vi "1D_array_from_binary_data.vi"(5 "little-endian?":bool, 7 "inputArray(type)":variant, 8 "error in (no error)":errorcluster, 11 "byteArray":u8[](array[numeric])) -> (0 "error out":errorcluster, 3 "dataArray":variant)   [LabVIEW 2015, in "BSON_convertors_Library.lvlib"]
uses:
  BSON_convertors_Library.lvlib
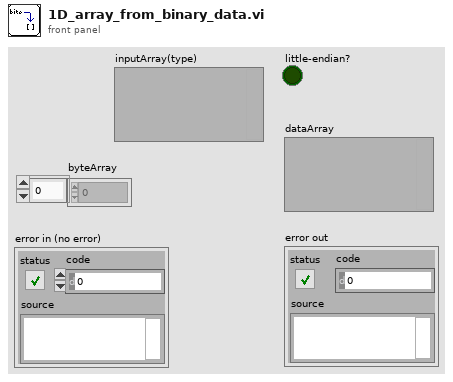
[diagram p1: front panel]
types:
  T1 = enum16{"big-endian, network order", "native, host order", "little-endian"}
  T2 = typedef "Type Descriptor Enumeration__ogtk.ctl" = enum8{"<Null>", "I8", "I16", "I32", "I64", "U8", "U16", "U32", "U64", "SGL", "DBL", "EXT", "CSG", "CDB", "CXT", "0x0F", "0x10", "0x11", "0x12", "0x13", "0x14", "Enum U8", "Enum U16", "Enum U32", "Enum U64", "SGL PQ", "DBL PQ", "EXT PQ", "CSG PQ", "CDB PQ", "CXT PQ", "0x1F", "0x20", "Boolean", "0x22", "0x23", "0x24", "0x25", "0x26", "0x27", "0x28", "0x29", "0x2A", "0x2B", "0x2C", "0x2D", "0x2E", "0x2F", "String", "0x31", "Path", "Pict", "0x34", "0x35", "0x36", "DAQ", "0x38", "0x39", "0x3A", "0x3B", "0x3C", "0x3D", "0x3E", "0x3F", "Array", "0x41", "0x42", "0x43", "0x44", "0x45", "0x46", "0x47", "0x48", "0x49", "0x4A", "0x4B", "0x4C", "0x4D", "0x4E", "0x4F", "Cluster", "0x51", "0x52", "Variant", "Waveform", "0x55", "0x56", "0x57", "0x58", "0x59", "0x5A", "0x5B", "0x5C", "0x5D", "0x5E", "0x5F", "0x60", "0x61", "0x62", "0x63", "0x64", "0x65", "0x66", "0x67", "0x68", "0x69", "0x6A", "0x6B", "0x6C", "0x6D", "0x6E", "0x6F", "Refnum"}
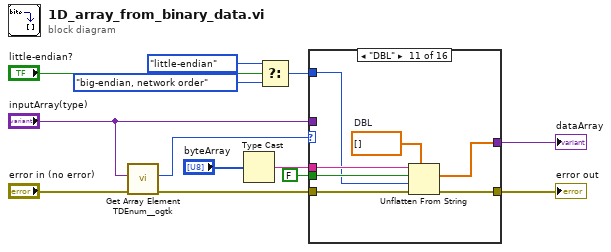
[diagram p0: block diagram]
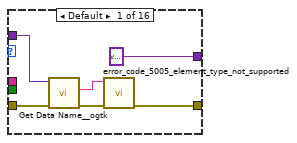
[diagram p2: hidden frame]
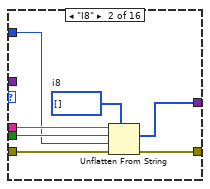
[diagram p3: hidden frame]
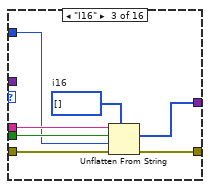
[diagram p4: hidden frame]
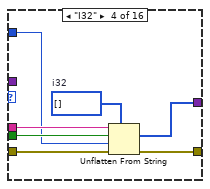
[diagram p5: hidden frame]
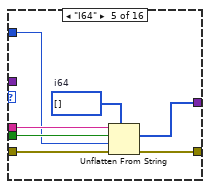
[diagram p6: hidden frame]
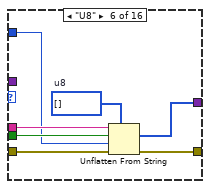
[diagram p7: hidden frame]
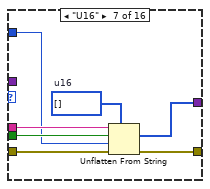
[diagram p8: hidden frame]
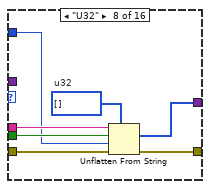
[diagram p9: hidden frame]
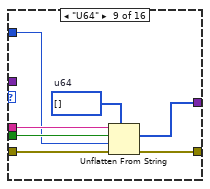
[diagram p10: hidden frame]
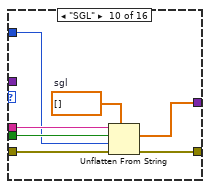
[diagram p11: hidden frame]
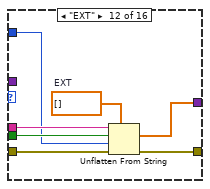
[diagram p12: hidden frame]
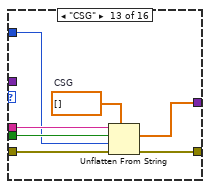
[diagram p13: hidden frame]
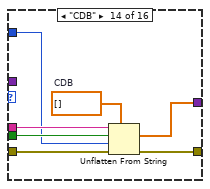
[diagram p14: hidden frame]
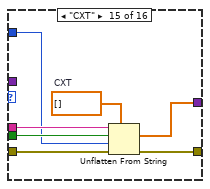
[diagram p15: hidden frame]
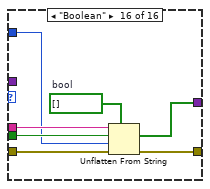
[diagram p16: hidden frame]
diagram:
  n1 = call <userlib>:"Get Array Element TDEnum__ogtk.vi"("error in (no error)"="error in (no error)", "Array"="inputArray(type)") -> ("error out"=w3:errorcluster, "Element Type"=w8:T2)  [unwired: 8 in]
  n2 = Type Cast(x="byteArray") -> (*(type *) &x=w5:string)  [unwired: 1 in]
  n3 = Select(t=T1."little-endian" ("byte order (0:big-endian, network order)"), s="little-endian?", f=T1."big-endian, network order" ("byte order (0:big-endian, network order)")) -> (s? t:f=w13:T1)
  n4 = case shown="\"DBL\"" w8 {
    tunnel: "inputArray(type)" -> [w19 _ _ _ _ _ _ _ _ _ _ _ _ _ _ _]
    tunnel: [w16 w20 w27 w34 w41 w48 w55 w62 w69 w76 w83 w90 w97 w104 w111 w118] -> w9
    tunnel: w13 -> [_ w24 w31 w38 w45 w52 w59 w66 w73 w80 w87 w94 w101 w108 w115 w122]
    tunnel: w5 -> [_ w26 w33 w40 w47 w54 w61 w68 w75 w82 w89 w96 w103 w110 w117 w124]
    tunnel: FALSE ("data includes array or string size? (T)") -> [_ w25 w32 w39 w46 w53 w60 w67 w74 w81 w88 w95 w102 w109 w116 w123]
    tunnel: w3 -> [w15 w23 w30 w37 w44 w51 w58 w65 w72 w79 w86 w93 w100 w107 w114 w121]
    tunnel: [variant ("Variant") w21 w28 w35 w42 w49 w56 w63 w70 w77 w84 w91 w98 w105 w112 w119] -> w2
    frame Default {
      n5 = call <userlib>:"Get Data Name__ogtk.vi"("error in (no error)"=w15, "Data"=w19) -> ("error out"=w17:errorcluster, "Data Name"=w18:string)  [unwired: 7 in, 1 out]
      n6 = call "error_code_5005_element_type_not_supported.vi"("error in (no error)"=w17, "name"=w18) -> ("error out"=w16:errorcluster)  [unwired: 9 in]
    }
    frame "I8" {
      w22 = i8[] []  # i8
      n7 = Unflatten From String(type=w22, binary string=w26, data includes array or string size? (T)=w25, byte order (0:big-endian, network order)=w24, error in (no error)=w23) -> (value=w21:i8[], error out=w20:errorcluster)  [unwired: 1 out]
    }
    frame "I16" {
      w29 = i16[] []  # i16
      n8 = Unflatten From String(type=w29, binary string=w33, data includes array or string size? (T)=w32, byte order (0:big-endian, network order)=w31, error in (no error)=w30) -> (value=w28:i16[], error out=w27:errorcluster)  [unwired: 1 out]
    }
    frame "I32" {
      w36 = i32[] []  # i32
      n9 = Unflatten From String(type=w36, binary string=w40, data includes array or string size? (T)=w39, byte order (0:big-endian, network order)=w38, error in (no error)=w37) -> (value=w35:i32[], error out=w34:errorcluster)  [unwired: 1 out]
    }
    frame "I64" {
      w43 = i64[] []  # i64
      n10 = Unflatten From String(type=w43, binary string=w47, data includes array or string size? (T)=w46, byte order (0:big-endian, network order)=w45, error in (no error)=w44) -> (value=w42:i64[], error out=w41:errorcluster)  [unwired: 1 out]
    }
    frame "U8" {
      w50 = u8[] []  # u8
      n11 = Unflatten From String(type=w50, binary string=w54, data includes array or string size? (T)=w53, byte order (0:big-endian, network order)=w52, error in (no error)=w51) -> (value=w49:u8[], error out=w48:errorcluster)  [unwired: 1 out]
    }
    frame "U16" {
      w57 = u16[] []  # u16
      n12 = Unflatten From String(type=w57, binary string=w61, data includes array or string size? (T)=w60, byte order (0:big-endian, network order)=w59, error in (no error)=w58) -> (value=w56:u16[], error out=w55:errorcluster)  [unwired: 1 out]
    }
    frame "U32" {
      w64 = u32[] []  # u32
      n13 = Unflatten From String(type=w64, binary string=w68, data includes array or string size? (T)=w67, byte order (0:big-endian, network order)=w66, error in (no error)=w65) -> (value=w63:u32[], error out=w62:errorcluster)  [unwired: 1 out]
    }
    frame "U64" {
      w71 = u64[] []  # u64
      n14 = Unflatten From String(type=w71, binary string=w75, data includes array or string size? (T)=w74, byte order (0:big-endian, network order)=w73, error in (no error)=w72) -> (value=w70:u64[], error out=w69:errorcluster)  [unwired: 1 out]
    }
    frame "SGL" {
      w78 = sgl[] []  # sgl
      n15 = Unflatten From String(type=w78, binary string=w82, data includes array or string size? (T)=w81, byte order (0:big-endian, network order)=w80, error in (no error)=w79) -> (value=w77:sgl[], error out=w76:errorcluster)  [unwired: 1 out]
    }
    frame "DBL" {
      w85 = dbl[] []  # DBL
      n16 = Unflatten From String(type=w85, binary string=w89, data includes array or string size? (T)=w88, byte order (0:big-endian, network order)=w87, error in (no error)=w86) -> (value=w84:dbl[], error out=w83:errorcluster)  [unwired: 1 out]
    }
    frame "EXT" {
      w92 = ext[] []  # EXT
      n17 = Unflatten From String(type=w92, binary string=w96, data includes array or string size? (T)=w95, byte order (0:big-endian, network order)=w94, error in (no error)=w93) -> (value=w91:ext[], error out=w90:errorcluster)  [unwired: 1 out]
    }
    frame "CSG" {
      w99 = csg[] []  # CSG
      n18 = Unflatten From String(type=w99, binary string=w103, data includes array or string size? (T)=w102, byte order (0:big-endian, network order)=w101, error in (no error)=w100) -> (value=w98:csg[], error out=w97:errorcluster)  [unwired: 1 out]
    }
    frame "CDB" {
      w106 = cdb[] []  # CDB
      n19 = Unflatten From String(type=w106, binary string=w110, data includes array or string size? (T)=w109, byte order (0:big-endian, network order)=w108, error in (no error)=w107) -> (value=w105:cdb[], error out=w104:errorcluster)  [unwired: 1 out]
    }
    frame "CXT" {
      w113 = cxt[] []  # CXT
      n20 = Unflatten From String(type=w113, binary string=w117, data includes array or string size? (T)=w116, byte order (0:big-endian, network order)=w115, error in (no error)=w114) -> (value=w112:cxt[], error out=w111:errorcluster)  [unwired: 1 out]
    }
    frame "Boolean" {
      w120 = bool[] []  # bool
      n21 = Unflatten From String(type=w120, binary string=w124, data includes array or string size? (T)=w123, byte order (0:big-endian, network order)=w122, error in (no error)=w121) -> (value=w119:bool[], error out=w118:errorcluster)  [unwired: 1 out]
    }
  }
  "error out" <- w9
  "dataArray" <- w2
